vi "TestOderProtokollUI_interface.vi"(10 "VI Refnum":refnum<vi>, 11 "Daten":T1={"Report.lvclass"=refnum, "Norm"="", "last State"=enum."Initialize", "Norm ID"=0, "parameter"=[], "EMTestCWS500N.lvclass"=refnum, "CEG4500.lvclass"=refnum, "Tektronix RSA5106A.lvclass"=refnum, "erfolgreich"=FALSE, "log"="", "Kommentar"="", "Device Enum"=enum."emTestCWS500N", "Test Enum"=enum."HF-Felder", "debug"=FALSE, "tab"=enum."Hauptmenü", "ESD Pistol.lvclass"=refnum, "SubPnl Refnum"=refnum, "TabCtl Refnum"=refnum, "ButtonsEinblenden?"=FALSE, "VKey"=enum."ASCII"}) -> (2 "TestMitGerät?":bool=TRUE, 3 "Daten out":T1={"Report.lvclass"=refnum, "Norm"="", "last State"=enum."Initialize", "Norm ID"=0, "parameter"=[], "EMTestCWS500N.lvclass"=refnum, "CEG4500.lvclass"=refnum, "Tektronix RSA5106A.lvclass"=refnum, "erfolgreich"=FALSE, "log"="", "Kommentar"="", "Device Enum"=enum."emTestCWS500N", "Test Enum"=enum."HF-Felder", "debug"=FALSE, "tab"=enum."Hauptmenü", "ESD Pistol.lvclass"=refnum, "SubPnl Refnum"=refnum, "TabCtl Refnum"=refnum, "ButtonsEinblenden?"=FALSE, "VKey"=enum."ASCII"})   [LabVIEW 2013]
uses:
  Main/controls/Data.ctl
  classes/Datastructure/Report/Report.lvclass
  classes/Devices/emTestCWS500N/EMTestCWS500N.lvclass
  classes/Devices/CEG4500/CEG4500.lvclass
  classes/Devices/Tektronix RSA5106A/Tektronix RSA5106A.lvclass
  ESD Pistol.lvclass
  Main/controls/State.ctl
  classes/Devices/DeviceInterface/Devices.ctl
  classes/Tests/TestInterface/Tests.ctl
  Tabs.ctl
  <vilib>/event_ctls.llb/eventvkey.ctl
panel:
  out "error out":errorcluster
  in  "error in (no error)":errorcluster
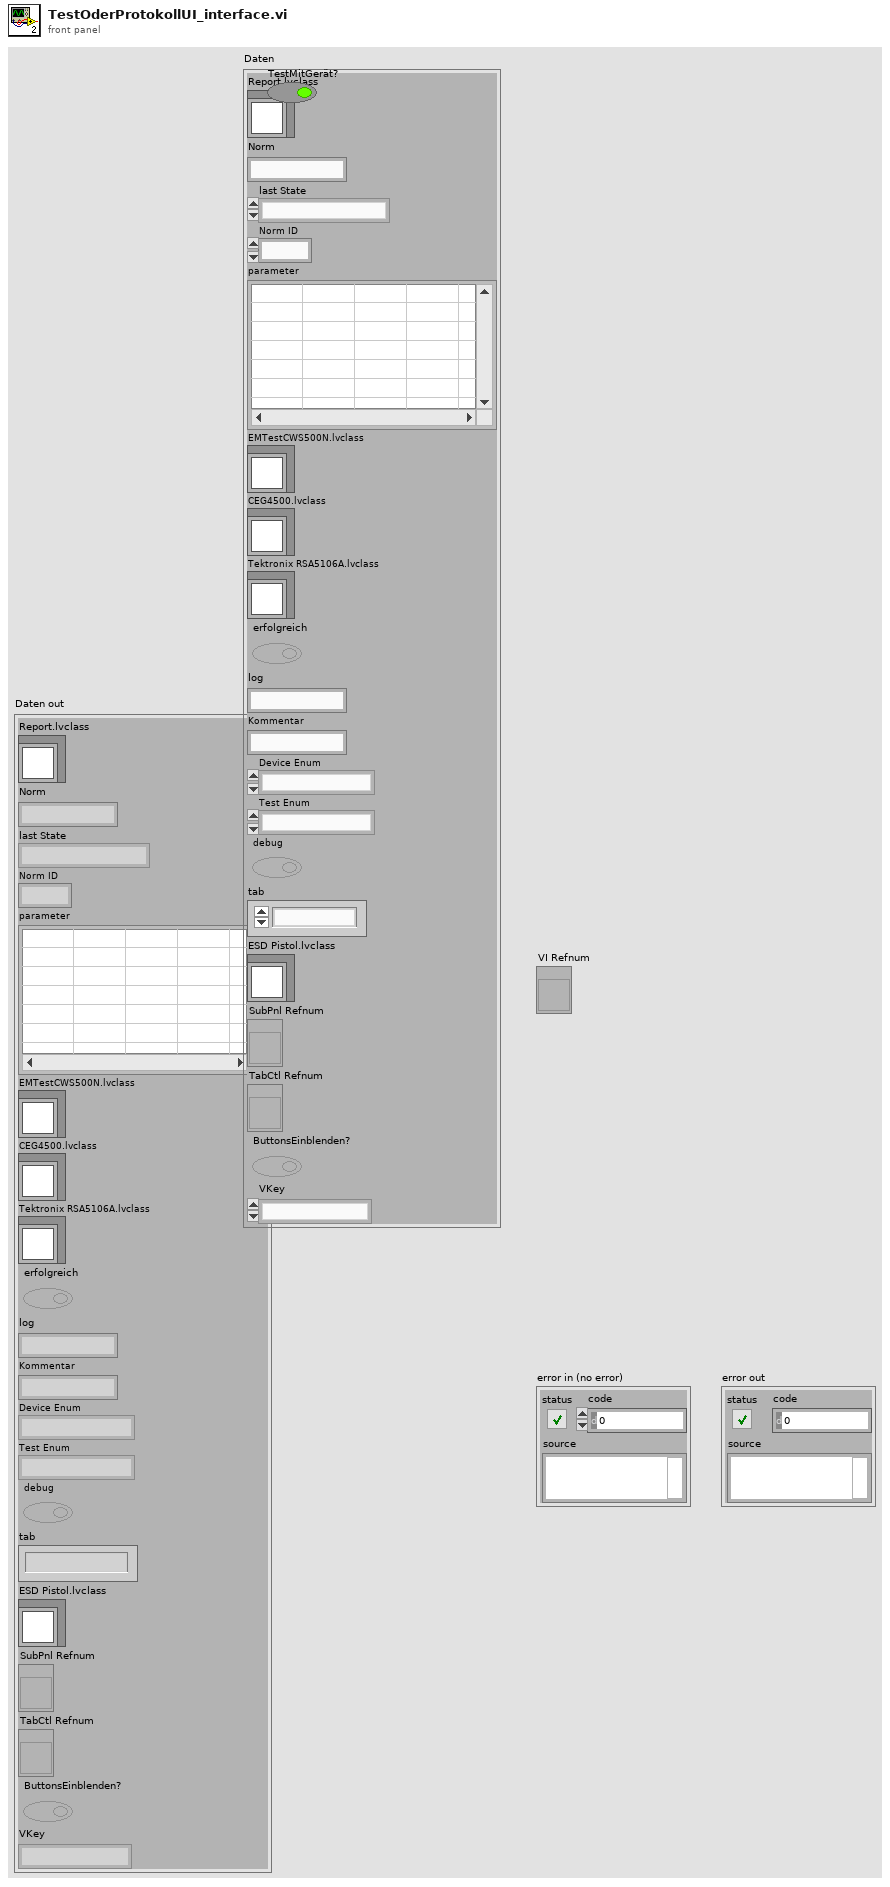
[diagram p1: front panel]
types:
  T1 = typedef "Data.ctl" = cluster{"Report.lvclass":refnum<class "Report.lvclass">, "Norm":string, "last State":T2, "Norm ID":i32, "parameter":string[][], "EMTestCWS500N.lvclass":refnum<class "EMTestCWS500N.lvclass">, "CEG4500.lvclass":refnum<class "CEG4500.lvclass">, "Tektronix RSA5106A.lvclass":refnum<class "Tektronix RSA5106A.lvclass">, "erfolgreich":bool, "log":string, "Kommentar":string, "Device Enum":T3, "Test Enum":T4, "debug":bool, "tab":T5, "ESD Pistol.lvclass":refnum<class "ESD Pistol.lvclass">, "SubPnl Refnum":refnum<vi>, "TabCtl Refnum":refnum<vi>, "ButtonsEinblenden?":bool, "VKey":T6}
  T2 = typedef "State.ctl" = enum16{"create Pdf", "edit Report", "load Report", "save Report", "do Test", "CDN Kalibrierung", "enter Report Parameters", "new Test", "Protokoll", "read Tree", "update Tree", "Fehler", "Initialize", "Wait for Event", "Exit"}
  T3 = typedef "Devices.ctl" = enum16{"unbekannt", "ESD Pistol", "Tektronix RSA5106A", "emTestCWS500N", "CEG-4500"}
  T4 = typedef "Tests.ctl" = enum16{"unbekannt", "Störaussendung", "Burst", "ESD", "Surge", "Spannungseinbruch", "HF-Felder"}
  T5 = typedef "Tabs.ctl" = enum32{"Hauptmenü", "Prüfbericht", "Einstellungen"}
  T6 = typedef "eventvkey.ctl" = enum16{"ASCII", "Enter", "Return", "Shift", "Ctrl", "Alt", "Cmd", "Opt", "Caps", "NumLock", "Clear", "Break", "Up", "Down", "Left", "Right", "Insert", "Delete", "Home", "End", "PageUp", "PageDown", "Escape", "Help", "Pause", "ScrollLock", "F1", "F2", "F3", "F4", "F5", "F6", "F7", "F8", "F9", "F10", "F11", "F12", "F13", "F14", "F15", "F16", "F17", "F18", "F19", "F20", "F21", "F22", "F23", "F24", "Play", "VolumeUp", "VolumeDown", "Mute", "Two Byte Char"}
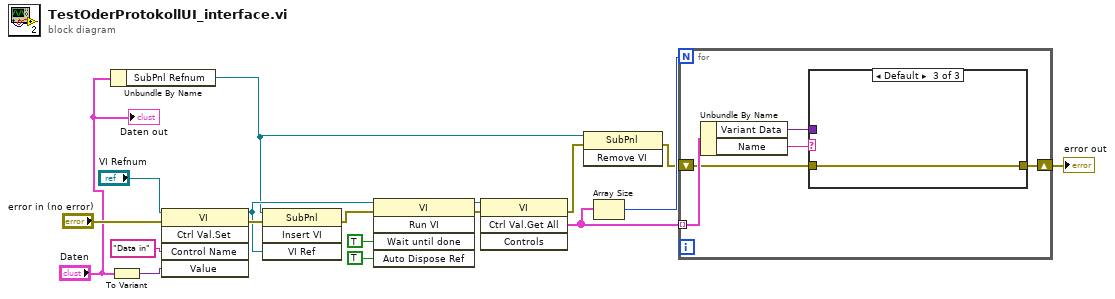
[diagram p0: block diagram]
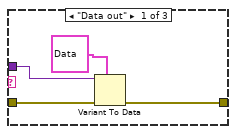
[diagram p2: hidden frame]
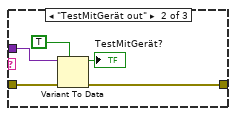
[diagram p3: hidden frame]
diagram:
  n1 = Unbundle By Name("Daten") -> ("SubPnl Refnum"=w2:refnum<vi>)
  n2 = To Variant(anything="Daten") -> (Variant=w8:variant)
  n3 = invoke class="VI" method="Ctrl Val.Set"(reference="VI Refnum", error in="error in (no error)", "Control Name"="Data in", "Value"=w8) -> (reference out=w3:refnum<vi>, error out=w4:errorcluster)  [unwired: 1 in, 3 out]
  n4 = invoke on="Invoke Node" class="SubPnl" method="Insert VI"(reference=w2, error in=w4, "VI Ref"=w3) -> (error out=w16:errorcluster)  [unwired: 1 in, 3 out]
  n5 = invoke on="Methodenknoten" class="VI" method="Run VI"(reference=w3, error in=w16, "Wait until done"=TRUE ("Warten bis beendet"), "Auto Dispose Ref"=TRUE ("Referenz automatisch schließen")) -> (reference out=w18:refnum<vi>, error out=w17:errorcluster)  [unwired: 1 in, 3 out]
  n6 = invoke class="VI" method="Ctrl Val.Get All"(reference=w18, error in=w17) -> (error out=w11:errorcluster, "Get All Control Values Variant"=w13:cluster{"Name":string, "Variant Data":variant}[])  [unwired: 2 in, 2 out]
  n7 = invoke on="Invoke Node" class="SubPnl" method="Remove VI"(reference=w2, error in=w11) -> (error out=w10:errorcluster)  [unwired: 1 in, 2 out]
  n8 = Array Size(array=w13) -> (size(s)=w12:i32)
  n9 = for {
    N: w12 -> [_]
    tunnel: w13 -> [w23] mode=indexing
    shift-right: [w19] -> w9
    shift-left: w10 -> [w20]
    n10 = Unbundle By Name(w23) -> ("Variant Data"=w21:variant, "Name"=w22:string)
    n11 = case shown="Default" w22 {
      tunnel: w21 -> [w27 w32 _]
      tunnel: w20 -> [w26 w31 w33]
      tunnel: [w25 w30 w33] -> w19
      frame "Data out" {
        n12 = Variant To Data(error in=w26, type=T1 {"Report.lvclass"=refnum, "Norm"="", "last State"=enum."create Pdf", "Norm ID"=0, "parameter"=[], "EMTestCWS500N.lvclass"=refnum, "CEG4500.lvclass"=refnum, "Tektronix RSA5106A.lvclass"=refnum, "erfolgreich"=FALSE, "log"="", "Kommentar"="", "Device Enum"=enum."unbekannt", "Test Enum"=enum."unbekannt", "debug"=FALSE, "tab"=enum."Hauptmenü", "ESD Pistol.lvclass"=refnum, "SubPnl Refnum"=refnum, "TabCtl Refnum"=refnum, "ButtonsEinblenden?"=FALSE, "VKey"=enum."ASCII"} ("Daten 2"), Variant=w27) -> (error out=w25:errorcluster)  [unwired: 1 out]
      }
      frame "TestMitGerät out" {
        n13 = Variant To Data(error in=w31, type=TRUE ("Boolean"), Variant=w32) -> (data=→"TestMitGerät?":bool, error out=w30:errorcluster)
      }
      frame Default {
      }
    }
  }
  "error out" <- w9
  "Daten out" <- "Daten"
